vi "Start-Stop Mask Test.vi"(8 "error in (no error)":errorcluster, 10 "Mask Test (T: Start)":bool=TRUE, 11 "VISA resource name":refnum<visa-resource-name>) -> (0 "error out":errorcluster, 3 "VISA resource name out":refnum<visa-resource-name>)   [LabVIEW 2020, in "Agilent 90000 Series.lvlib"]
doc: "Starts and stops a mask test."
uses:
  Agilent 90000 Series.lvlib
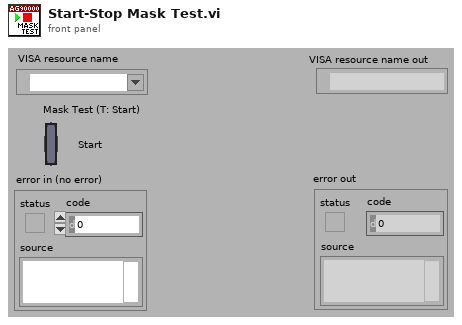
[diagram p1: front panel]
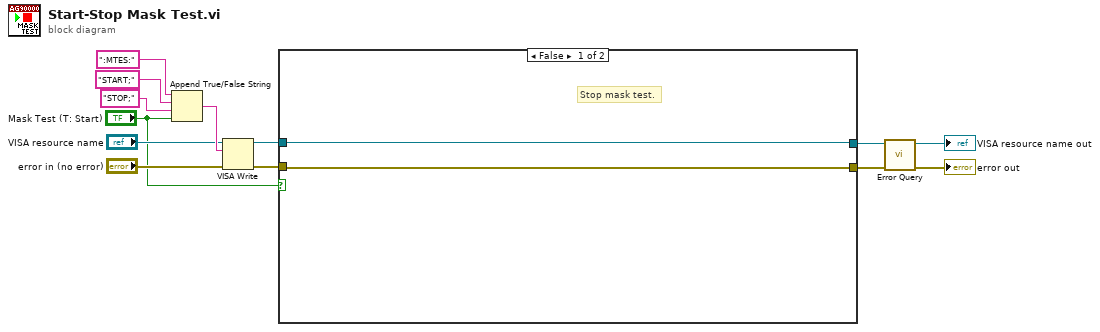
[diagram p0: block diagram]
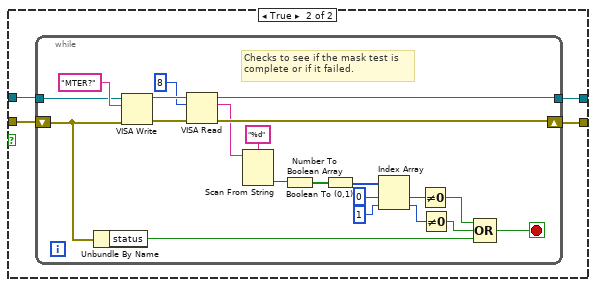
[diagram p2: hidden frame]
diagram:
  n1 = Append True/False String(1:"Mask Test (T: Start)", 2:"STOP;" ("false string"), 3:"START;" ("true string"), 4:":MTES:" ("string (\"\")")) -> (0:w10:string)
  n2 = VISA Write(VISA resource name="VISA resource name", write buffer=w10, error in (no error)="error in (no error)") -> (VISA resource name out=w7:refnum<visa-resource-name>, error out=w6:errorcluster)  [unwired: 1 out]
  n3 = case shown="False" "Mask Test (T: Start)" {
    tunnel: [w15 w19] -> w4
    tunnel: [w14 w18] -> w3
    tunnel: w7 -> [w15 w17]
    tunnel: w6 -> [w14 w16]
    frame False {
      # "Stop mask test."
    }
    frame True {
      n4 = while {
        tunnel: [w39] -> w19
        shift-right: [w40] -> w18
        shift-left: w16 -> [w20]
        tunnel: w17 -> [w27]
        stop <- w25 stop-if-true
        # "Checks to see if the mask test is \ncomplete or if it failed."
        n5 = Unbundle By Name(w20) -> ("status"=w22:bool)
        n6 = VISA Write(VISA resource name=w27, write buffer="MTER?", error in (no error)=w20) -> (VISA resource name out=w37:refnum<visa-resource-name>, error out=w36:errorcluster)  [unwired: 1 out]
        n7 = VISA Read(VISA resource name=w37, byte count=u32 8, error in (no error)=w36) -> (VISA resource name out=w39:refnum<visa-resource-name>, read buffer=w34:string, error out=w40:errorcluster)  [unwired: 1 out]
        n8 = Scan From String(format string="%d", input string=w34) -> (output 1=w29:i32)  [unwired: 2 in, 4 out]
        n9 = Number To Boolean Array(number=w29) -> (Boolean array=w32:bool[])
        n10 = Boolean To (0,1)(Boolean=w32) -> (0, 1=w31:i16[])
        n11 = Index Array(array=w31, index #1=0 ("index"), index #2=1 ("index")) -> (element #1=w28:i16, element #2=w23:i16)
        n12 = Not Equal To 0?(x=w28) -> (x != 0?=w26:bool)
        n13 = Not Equal To 0?(x=w23) -> (x != 0?=w21:bool)
        n14 = Compound Arithmetic op=OR(w26, w21, w22) -> (w25:bool)
      }
    }
  }
  n15 = call "Error Query.vi"("error in (no error)"=w3, "VISA resource name"=w4) -> ("error out"=→"error out":errorcluster, "VISA resource name out"=→"VISA resource name out":refnum<visa-resource-name>)  [unwired: 8 out]
